vi "example_GArrayUploadFile.vi"() -> ()   [LabVIEW 2021]
uses:
  <vilib>/Galil/resources/gclib/gclib.lvlib
  <vilib>/Galil/resources/gclibo/gclibo.lvlib
panel:
  in  "File Location":string="C:\\Program Files\\National Instruments\\LabVIEW 2021\\vi.lib\\Galil\\examples\\vi_examples\\example_files\\array_upload.csv"
  in  "Command":string="DM A[5]; A[0]=1; A[1]=2; A[2]=3; A[3]=4; A[4]=5"
  out "Error Out":errorcluster
  in  "IP Address":string="192.168.1.77"
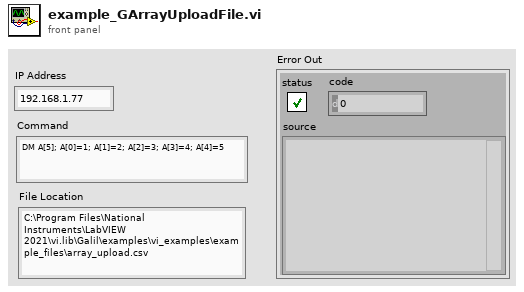
[diagram p1: front panel]
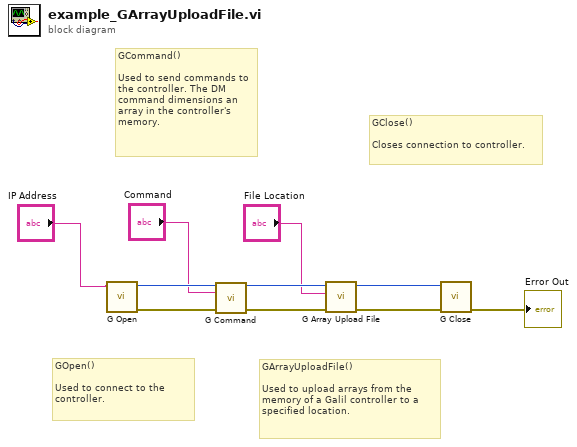
[diagram p0: block diagram]
diagram:
  # "GClose()\n\nCloses connection to controller."
  # "GArrayUploadFile()\n\nUsed to upload arrays from the memory of a Galil controller to a specified location."
  # "GCommand()\n\nUsed to send commands to the controller. The DM command dimensions an array in the controller's memory."
  # "GOpen()\n\nUsed to connect to the controller."
  n1 = call <vilib>:"G Open.vi"("address"="IP Address") -> ("error out"=w4:errorcluster, "g out"=w6:u64)  [unwired: 8 in]
  n2 = call <vilib>:"G Command.vi"("g"=w6, "command"="Command", "error in (no error)"=w4) -> ("g out"=w2:u64, "error out"=w3:errorcluster)  [unwired: 10 in, 1 out]
  n3 = call <vilib>:"G Array Upload File.vi"("error in (no error)"=w3, "file_path"="File Location", "g"=w2) -> ("error out"=w9:errorcluster, "g out"=w10:u64)  [unwired: 6 in]
  n4 = call <vilib>:"G Close.vi"("error in (no error)"=w9, "g"=w10) -> ("error out"=→"Error Out":errorcluster)  [unwired: 9 in]
